vi "IPC-Modbus-BitArrayToU8Array.vi"(10 "Bit Array":bool[](array[boolean]), 11 "U8 Array size":u8) -> (3 "U8 Array":u8[](array[numeric]))   [LabVIEW 2014]
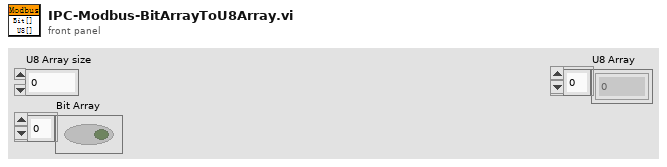
[diagram p1: front panel]
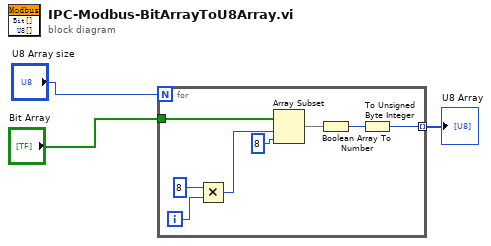
[diagram p0: block diagram]
diagram:
  n1 = for {
    N: "U8 Array size" -> [_]
    tunnel: "Bit Array" -> [w9]
    tunnel: [w4] -> w1 mode=indexing
    i -> [w11]
    n2 = Multiply(x=8, y=w11) -> (x*y=w8:i32)
    n3 = Array Subset(array=w9, index=w8, length=8 ("长度")) -> (w6:bool[])
    n4 = Boolean Array To Number(Boolean array=w6) -> (number=w5:u32)
    n5 = To Unsigned Byte Integer(number=w5) -> (unsigned 8bit integer=w4:u8)
  }
  "U8 Array" <- w1
